vi "DMA Constants.vi"() -> ()   [LabVIEW 2015]
panel:
  in  "L (m)":dbl=0.4444
  in  "r2 (m)":dbl=0.01958
  in  "r1 (m)":dbl=0.00937
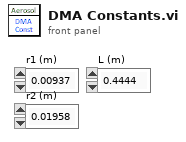
[diagram p1: front panel]
diagram:
